vi "GetXMLValueForTag.vi"(8 "error in (no error)":errorcluster, 9 "tag":string, 11 "XML":string) -> (0 "error out":errorcluster, 2 "Found?":bool, 3 "value":string)   [LabVIEW 2016, in "NI_NPW_Loading Project Info.lvlib"]
uses:
  <resource>/dialog/NewProjectWizard/Loading Project Info/NI_NPW_Loading Project Info.lvlib
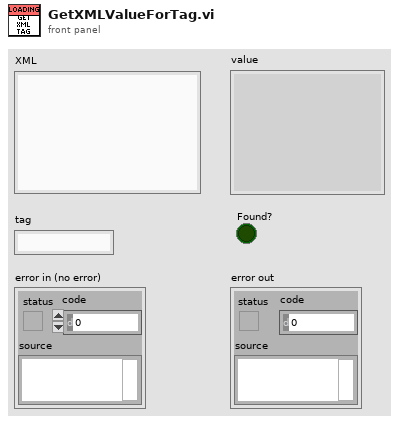
[diagram p1: front panel]
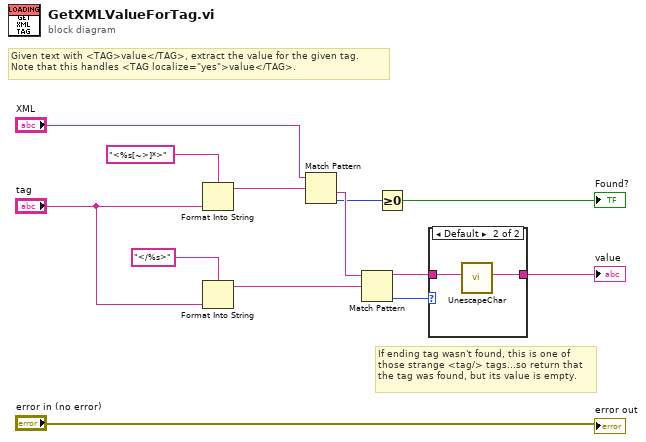
[diagram p0: block diagram]
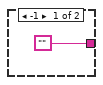
[diagram p2: hidden frame]
diagram:
  # "If ending tag wasn't found, this is one of\nthose strange <tag/> tags...so return that\nthe tag was found, but its value is empty."
  # "Given text with <TAG>value</TAG>, extract the value for the given tag.\nNote that this handles <TAG localize=\"yes\">value</TAG>."
  n1 = Format Into String(format string="<%s[~>]*>" ("regular expression"), "tag") -> (resulting string=w8:string)  [unwired: 2 in, 1 out]
  n2 = Format Into String(format string="</%s>" ("regular expression"), "tag") -> (resulting string=w7:string)  [unwired: 2 in, 1 out]
  n3 = Match Pattern(string="XML", regular expression=w8) -> (after substring=w13:string, offset past match=w3:i32)  [unwired: 1 in, 2 out]
  n4 = Match Pattern(string=w13, regular expression=w7) -> (before substring=w6:string, offset past match=w1:i32)  [unwired: 1 in, 2 out]
  n5 = Greater Or Equal To 0?(x=w3) -> (x >= 0?=→"Found?":bool)
  n6 = case shown="Default" w1 {
    tunnel: w6 -> [_ w16]
    tunnel: ["" w15] -> w4
    frame -1 {
    }
    frame Default {
      n7 = call <vilib>:"UnescapeChar.vi"("XML In"=w16) -> ("XML Out"=w15:string)  [unwired: 10 in]
    }
  }
  "value" <- w4
  "error out" <- "error in (no error)"
